vi "Manipulation2.vi"() -> ()   [LabVIEW 2017]
panel:
  in  "stop":bool
  in  "Combo Box":string(combo)
  out "Slide":dbl(slide) scale=0.0..10.0
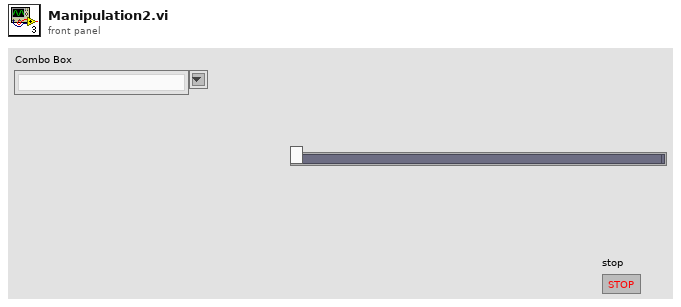
[diagram p1: front panel]
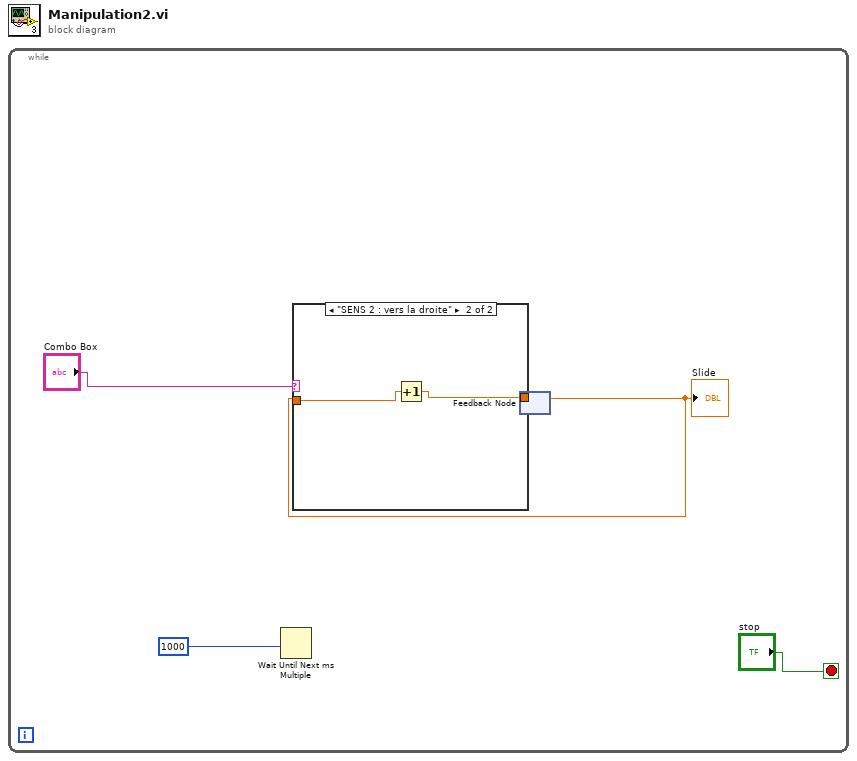
[diagram p0: block diagram]
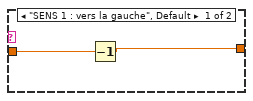
[diagram p2: hidden frame]
diagram:
  n1 = while {
    stop <- "stop" stop-if-true
    n2 = Wait Until Next ms Multiple(millisecond multiple=1000) -> ()  [unwired: 1 out]
    n3 = feedback #1() -> (w2:dbl)  [unwired: 1 in]
    "Slide" <- w2
    n4 = case shown="\"SENS 2 : vers la droite\"" "Combo Box" {
      tunnel: [w7 w9] -> w3
      tunnel: w2 -> [w6 w8]
      frame "SENS 1 : vers la gauche", Default {
        n5 = Decrement(x=w6) -> (x-1=w7:dbl)
      }
      frame "SENS 2 : vers la droite" {
        n6 = Increment(x=w8) -> (x+1=w9:dbl)
      }
    }
    n7 = feedback-in #1(w3) -> ()
  }
